vi "Run Filter.vi"(8 "error in (no error)":errorcluster, 10 "resource entries in":T1[](array[typedef]) {"FPGA CD Ref" format="%.0x"; "reserver" format="%.0x"}, 11 "Resource Name Filter in":refnum<class "Resource Name Filter.lvclass">) -> (0 "error out":errorcluster, 2 "resource entries out":T1[](array[typedef]) {"FPGA CD Ref" format="%.0x"; "reserver" format="%.0x"})   [LabVIEW 2016, in "FPGA Resource Manager System Definition.lvlib" / "Resource Name Filter.lvclass"]
uses:
  Resource Name Filter.lvclass
  resource info.ctl
  <vilib>/NI Veristand/Custom Device API/Custom Device Item Ref.ctl
  Resource Name Filter.lvclass/Resource Name Filter.ctl
  <vilib>/NI VeriStand/Custom Device API/Custom Device API.lvlib
  FPGA Resource Manager System Definition.lvlib
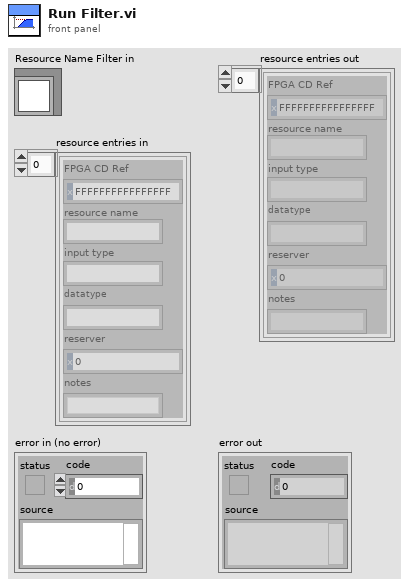
[diagram p1: front panel]
types:
  T1 = typedef "FPGA Resource Manager System Definition.lvlib/resource info.ctl" = cluster{"FPGA CD Ref":T2, "resource name":string, "input type":string, "datatype":string, "reserver":T2, "notes":string}
  T2 = typedef "Custom Device API.lvlib/Custom Device Item Ref.ctl" = u64
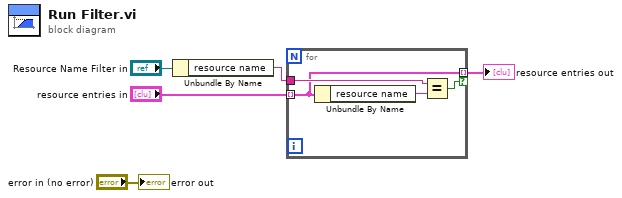
[diagram p0: block diagram]
diagram:
  n1 = Unbundle By Name("Resource Name Filter in") -> ("resource name"=w3:string)
  n2 = for {
    tunnel: "resource entries in" -> [w6] mode=indexing
    tunnel: w3 -> [w8]
    tunnel: [w6] -> w2 mode=indexing if=w7
    n3 = Unbundle By Name(w6) -> ("resource name"=w9:string)
    n4 = Equal?(x=w8, y=w9) -> (x = y?=w7:bool)
  }
  "resource entries out" <- w2
  "error out" <- "error in (no error)"
